vi "例子.vi"   [LabVIEW 2016]
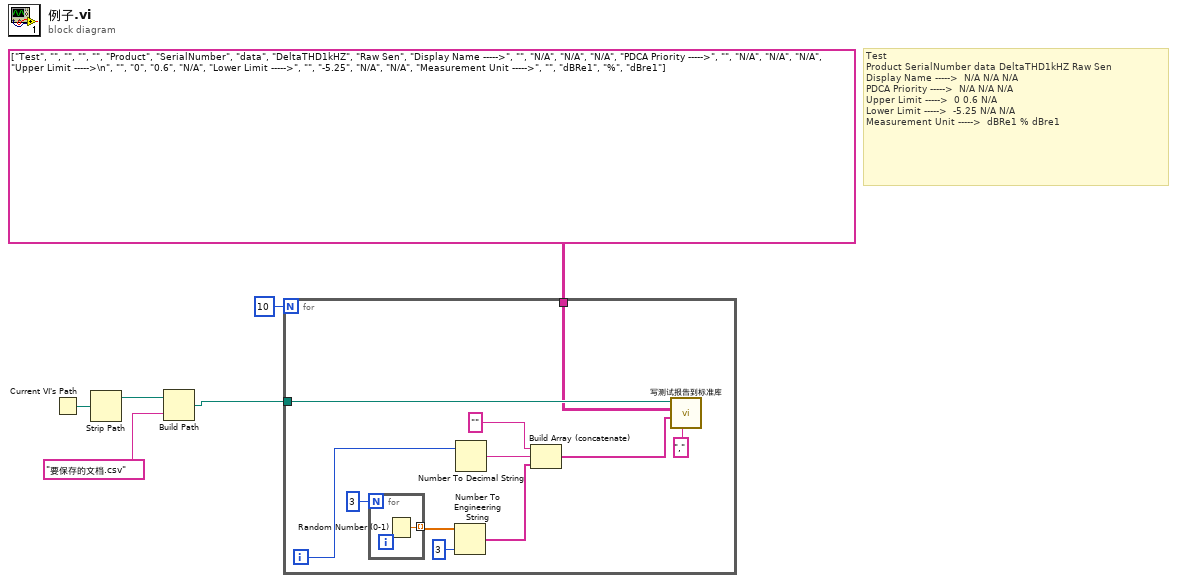
[diagram p0: block diagram]
diagram:
  # "Test\t\t\t\t\nProduct\tSerialNumber\tdata\tDeltaTHD1kHZ\tRaw Sen\nDisplay Name ----->\t\tN/A\tN/A\tN/A\nPDCA Priority ----->\t\tN/A\tN/A\tN/A\nUpper Limit ----->\t\t0\t0.6\tN/A\nLower Limit ----->\t\t-5.25\tN/A\tN/A\nMeasurement Unit ----->\t\tdBRe1\t%\tdBre1"
  n1 = Current VI's Path() -> (path=w6:path)
  n2 = Strip Path(path=w6) -> (stripped path=w5:path)  [unwired: 1 out]
  n3 = Build Path(base path=w5, name or relative path="要保存的文档.csv" ("名称或相对路径")) -> (appended path=w2:path)
  n4 = for {
    N: 10 -> [_]
    tunnel: w2 -> [w17]
    tunnel: string[][] [["Test", "", "", "", ""], ["Product", "SerialNumber", "data", "DeltaTHD1kHZ", "Raw Sen"], ["Display Name ----->", "", "N/A", "N/A", "N/A"], ["PDCA Priority ----->", "", "N/A", "N/A", "N/A"], ["Upper Limit ----->\n", "", "0", "0.6", "N/A"], ["Lower Limit ----->", "", "-5.25", "N/A", "N/A"], ["Measurement Unit ----->", "", "dBRe1", "%", "dBre1"]] ("表头") -> [w16]
    i -> [w15]
    n5 = for {
      N: 3 -> [_]
      tunnel: [w18] -> w13 mode=indexing
      n6 = Random Number (0-1)() -> (number: 0 to 1=w18:dbl)
    }
    n7 = Number To Engineering String(2:i16 3 ("精度(6)"), 4:w13) -> (0:w11:string[])  [unwired: 2 in]
    n8 = Number To Decimal String(number=w15) -> (decimal integer string=w10:string)  [unwired: 1 in]
    n9 = Build Array (concatenate)("", w10, w11) -> (w8:string[])
    n10 = call "写测试报告到标准库.vi"("delimiter (\\t)"="," ("delimiter (\\t)"), "1D data"=w8, "表头"=w16, "写入配置文件地址"=w17) -> ()  [unwired: 8 in]
  }
